vi "Renew UI Attributes From Configuration.vi"(8 "error in (no error)":errorcluster, 11 "ScriptsConfiguration in":refnum<class "ScriptSetting.lvclass">) -> (0 "error out":errorcluster, 3 "ScriptsConfiguration out":refnum<class "ScriptSetting.lvclass">)   [LabVIEW 2015, in "ScriptSetting.lvclass"]
uses:
  ScriptSetting.lvclass
  ScriptSetting.lvclass/ScriptSetting.ctl
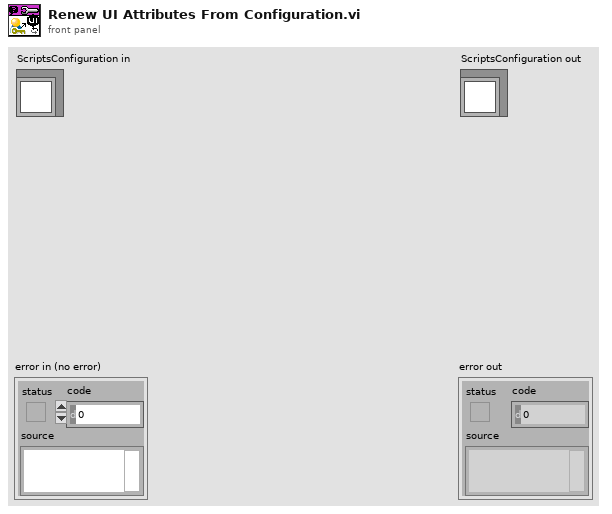
[diagram p1: front panel]
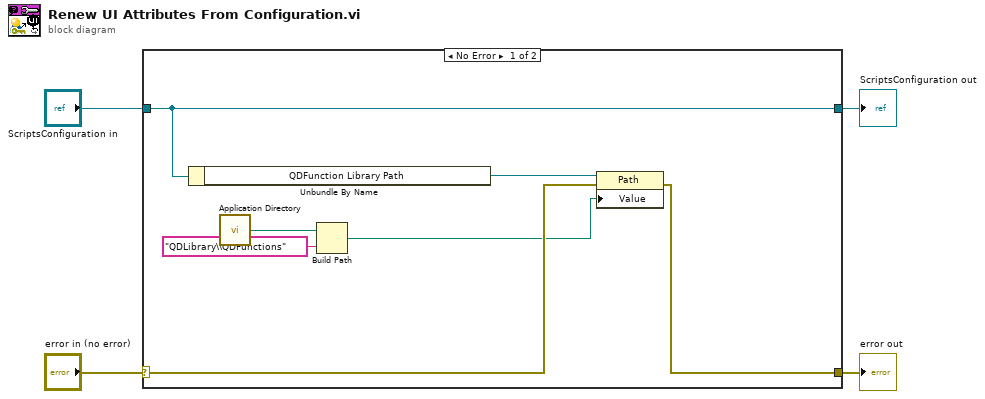
[diagram p0: block diagram]
diagram:
  n1 = case shown="No Error" "error in (no error)" {
    selector: "error in (no error)" -> [w7 w13]
    tunnel: [w5 w13] -> w3
    tunnel: [w9 w12] -> w1
    tunnel: "ScriptsConfiguration in" -> [w9 w12]
    frame No Error {
      n2 = Unbundle By Name(w9) -> ("QDFunction Library Path"=w8:refnum<vi>)
      n3 = call <vilib>:"Application Directory.vi"() -> ("Application Directory"=w11:path)
      n4 = Build Path(base path=w11, name or relative path="QDLibrary\\QDFunctions") -> (appended path=w6:path)
      n5 = property class="Path"(reference=w8, error in=w7, "Value"=w6) -> (error out=w5:errorcluster)  [unwired: 1 out]
    }
    frame Error {
    }
  }
  "error out" <- w3
  "ScriptsConfiguration out" <- w1
